vi "Determine Generation Type from File.vi"(8 "error in (no error)":errorcluster, 11 "cfg file":path) -> (0 "error out":errorcluster, 3 "output type":T1 caption="generation type")   [LabVIEW 2021]
uses:
  controls/generation type.ctl
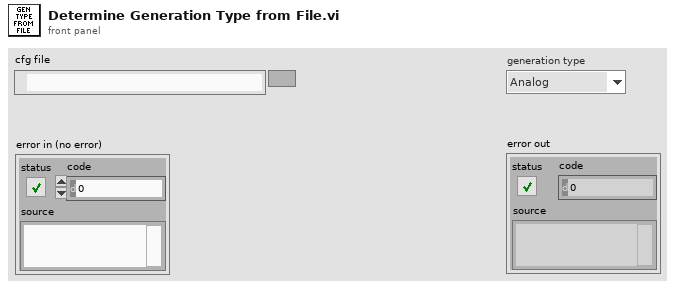
[diagram p1: front panel]
types:
  T1 = typedef "generation type.ctl" = enum32{"Analog", "Digital Serial"}
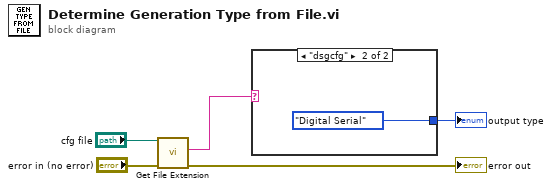
[diagram p0: block diagram]
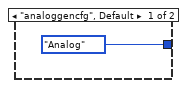
[diagram p2: hidden frame]
diagram:
  n1 = call <vilib>:"Get File Extension.vi"("error in (no error)"="error in (no error)", "file"="cfg file") -> ("error out"=→"error out":errorcluster, "lowercase file extension"=w2:string)  [unwired: 5 in, 3 out]
  n2 = case shown="\"dsgcfg\"" w2 {
    tunnel: [generation_type."Analog" ("output type") generation_type."Digital Serial" ("output type")] -> w1
    frame "analoggencfg", Default {
    }
    frame "dsgcfg" {
    }
  }
  "output type" <- w1
